vi "Field Info to Cluster Item Info (Scalar).vi"(1 "Table Info":T3) -> (0 "Cluster Item":T1={"Label.Text"="", "Type"=enum."Invalid Type", "Default Value"=variant(string ""), "Description"=""})   [LabVIEW 2021]
uses:
  edt.lib/sqlite.lib/SQLite Field Info.ctl
  edt.lib/sqlite.lib/SQLite Data Type.ctl
  edt.lib/vi_script.lib/Cluster Item Info.ctl
  <vilib>/Utility/Data Type/Type Definitions/Data Type.ctl
  SQLite Data Type to LV Data Type.ctl
  <vilib>/Utility/Data Type/NI_Data Type.lvlib
  edt.lib/vi_script.lib/EDT VI Script.lvlib
  edt.lib/sqlite.lib/EDT SQLite+.lvlib
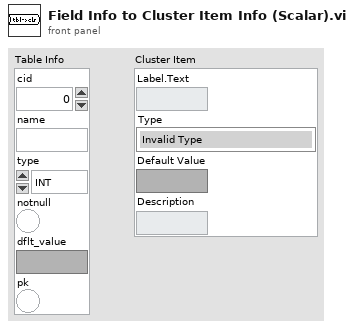
[diagram p1: front panel]
types:
  T1 = typedef "EDT VI Script.lvlib/Cluster Item Info.ctl" = cluster{"Label.Text":string, "Type":T2, "Default Value":variant, "Description":string}
  T2 = typedef "NI_Data Type.lvlib/Data Type.ctl" = enum8{"Invalid Type", "Void", "I8", "I16", "I32", "I64", "U8", "U16", "U32", "U64", "Single Float", "Double Float", "Extended Float", "Single Complex", "Double Complex", "Extended Complex", "Enum U8", "Enum U16", "Enum U32", "Enum U64", "Single Float With Unit", "Double Float With Unit", "Extended Float With Unit", "Single Complex with Unit", "Double Complex with Unit", "Extended Complex with Unit", "Boolean", "String", "Path", "Picture", "Tag", "Array", "Cluster", "Variant", "LV Variant", "Waveform", "Timestamp", "Digital Waveform", "Digital Data", "ExpressData", "Refnum", "External Data", "VI", "Poly VI", "LabVIEW Class Instance", "Fixed Point", "Set Collection", "Map Collection"}
  T3 = typedef "EDT SQLite+.lvlib/SQLite Field Info.ctl" = cluster{"cid":i32, "name":string, "type":T4, "notnull":bool, "dflt_value":variant, "pk":bool}
  T4 = typedef "EDT SQLite+.lvlib/SQLite Data Type.ctl" = enum16{"INT", "INTEGER", "TINYINT", "SMALLINT", "MEDIUMINT", "BIGINT", "UNSIGNED BIG INT", "INT2", "INT8", "CHARACTER", "VARCHAR", "VARYING CHARACTER", "NCHAR", "NATIVE CHARACTER", "NVARCHAR", "TEXT", "CLOB", "BLOB", "no datatype specified", "REAL", "DOUBLE", "DOUBLE PRECISION", "FLOAT", "NUMERIC", "DECIMAL", "BOOLEAN", "DATE", "DATETIME"}
  T5 = typedef "SQLite Data Type to LV Data Type.ctl" = map{T4, T2}
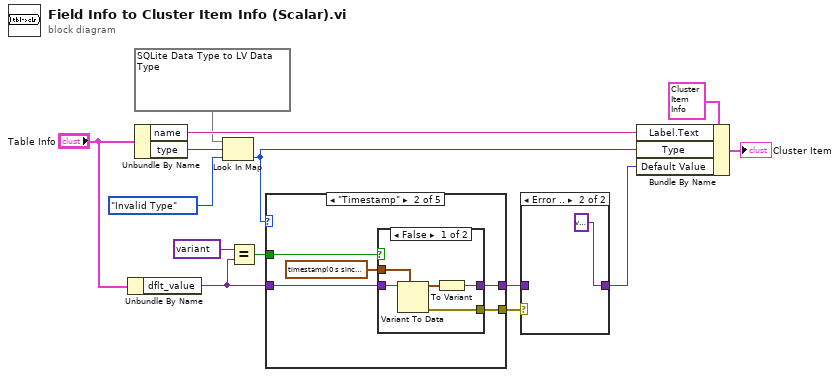
[diagram p0: block diagram]
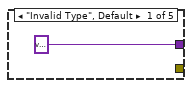
[diagram p3: hidden frame]
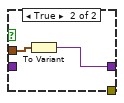
[diagram p4: hidden frame]
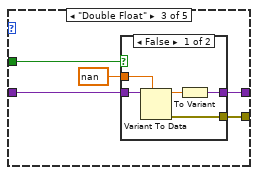
[diagram p5: hidden frame]
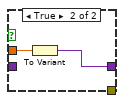
[diagram p6: hidden frame]
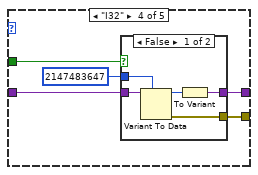
[diagram p7: hidden frame]
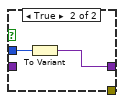
[diagram p8: hidden frame]
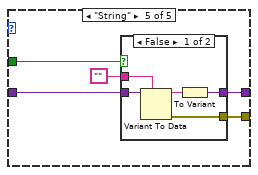
[diagram p9: hidden frame]
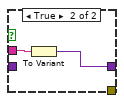
[diagram p10: hidden frame]
diagram:
  n1 = Unbundle By Name("Table Info") -> ("dflt_value"=w3:variant)
  n2 = Unbundle By Name("Table Info") -> ("name"=w9:string, "type"=w7:T4)
  n3 = Look In Map(map=T5 {enum."INT"=enum."I32", enum."INTEGER"=enum."I32", enum."TINYINT"=enum."I32", enum."SMALLINT"=enum."I32", enum."MEDIUMINT"=enum."I32", enum."BIGINT"=enum."I32", enum."UNSIGNED BIG INT"=enum."I32", enum."INT2"=enum."I32", enum."INT8"=enum."I32", enum."CHARACTER"=enum."String", enum."VARCHAR"=enum."String", enum."VARYING CHARACTER"=enum."String", enum."NCHAR"=enum."String", enum."NATIVE CHARACTER"=enum."String", enum."NVARCHAR"=enum."String", enum."TEXT"=enum."String", enum."CLOB"=enum."String", enum."BLOB"=enum."String", enum."no datatype specified"=enum."String", enum."REAL"=enum."Double Float", enum."DOUBLE"=enum."Double Float", enum."DOUBLE PRECISION"=enum."Double Float", enum."FLOAT"=enum."Double Float", enum."NUMERIC"=enum."Double Float", enum."DECIMAL"=enum."Double Float", enum."BOOLEAN"=enum."I32", enum."DATE"=enum."Timestamp", enum."DATETIME"=enum."Timestamp"} ("SQLite Data Type to LV Data Type"), key=w7, default value=Data_Type."Invalid Type" ("type")) -> (value=w5:T2)  [unwired: 1 out]
  n4 = Equal?(x=variant ("dflt_value"), y=w3) -> (x = y?=w1:bool)
  n5 = case shown="\"Timestamp\"" w5 {
    tunnel: w3 -> [_ w20 w32 w44 w56]
    tunnel: [variant ("Variant") w18 w31 w43 w55] -> w13
    tunnel: [_ w17 w29 w41 w53] -> w14
    tunnel: w1 -> [_ w16 w28 w40 w52]
    frame "Invalid Type", Default {
    }
    frame "Timestamp" {
      n6 = case shown="False" w16 {
        tunnel: [w24 w27] -> w18
        tunnel: w20 -> [w25 _]
        tunnel: timestamp(0 s since 1904-01-01) ("Time Stamp") -> [w22 w26]
        tunnel: [w21 _] -> w17
        frame False {
          n7 = Variant To Data(type=w22, Variant=w25) -> (data=w23:timestamp, error out=w21:errorcluster)  [unwired: 1 in]
          n8 = To Variant(anything=w23) -> (Variant=w24:variant)
        }
        frame True {
          n9 = To Variant(anything=w26) -> (Variant=w27:variant)
        }
      }
    }
    frame "Double Float" {
      n10 = case shown="False" w28 {
        tunnel: [w36 w39] -> w31
        tunnel: w32 -> [w37 _]
        tunnel: nan -> [w34 w38]
        tunnel: [w33 _] -> w29
        frame False {
          n11 = Variant To Data(type=w34, Variant=w37) -> (data=w35:dbl, error out=w33:errorcluster)  [unwired: 1 in]
          n12 = To Variant(anything=w35) -> (Variant=w36:variant)
        }
        frame True {
          n13 = To Variant(anything=w38) -> (Variant=w39:variant)
        }
      }
    }
    frame "I32" {
      n14 = case shown="False" w40 {
        tunnel: [w48 w51] -> w43
        tunnel: w44 -> [w49 _]
        tunnel: 2147483647 -> [w46 w50]
        tunnel: [w45 _] -> w41
        frame False {
          n15 = Variant To Data(type=w46, Variant=w49) -> (data=w47:i32, error out=w45:errorcluster)  [unwired: 1 in]
          n16 = To Variant(anything=w47) -> (Variant=w48:variant)
        }
        frame True {
          n17 = To Variant(anything=w50) -> (Variant=w51:variant)
        }
      }
    }
    frame "String" {
      n18 = case shown="False" w52 {
        tunnel: [w60 w63] -> w55
        tunnel: w56 -> [w61 _]
        tunnel: "" -> [w58 w62]
        tunnel: [w57 _] -> w53
        frame False {
          n19 = Variant To Data(type=w58, Variant=w61) -> (data=w59:string, error out=w57:errorcluster)  [unwired: 1 in]
          n20 = To Variant(anything=w59) -> (Variant=w60:variant)
        }
        frame True {
          n21 = To Variant(anything=w62) -> (Variant=w63:variant)
        }
      }
    }
  }
  n22 = case shown="Error .." w14 {
    tunnel: w13 -> [w64 _]
    tunnel: [w64 variant ("Variant")] -> w12
    frame No Error {
    }
    frame Error {
    }
  }
  n23 = Bundle By Name(cluster=T1 {"Label.Text"="", "Type"=enum."Invalid Type", "Default Value"=variant(string ""), "Description"=""} ("Cluster Item"), "Label.Text"=w9, "Type"=w5, "Default Value"=w12) -> (→"Cluster Item":T1)
